vi "Get Graph.vi"(8 "error in (no error)":errorcluster, 11 "IV in":refnum<class "IV.lvclass">) -> (0 "error out":errorcluster, 1 "Y":dbl[](array[numeric]), 2 "X":dbl[](array[numeric]), 3 "IV out":refnum<class "IV.lvclass">, 4 "dY/dX":dbl[](array[numeric]))   [LabVIEW 2018, in "IV.lvclass"]
uses:
  IV.lvclass
  data/IV_data.lvclass
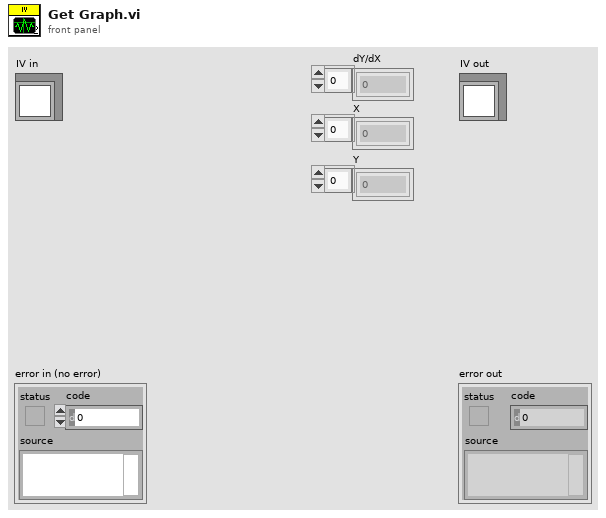
[diagram p1: front panel]
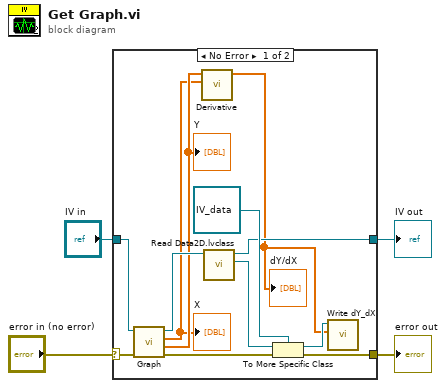
[diagram p0: block diagram]
diagram:
  n1 = case shown="No Error" "error in (no error)" {
    selector: "error in (no error)" -> [w14 w18]
    tunnel: [w6 w18] -> w3
    tunnel: [w10 w17] -> w1
    tunnel: "IV in" -> [w16 w17]
    frame No Error {
      n2 = call-dynamic "Graph.vi"("error in (no error)"=w14, "IV in"=w16) -> ("error out"=w15:errorcluster, "Y"=w9:dbl[], "X"=w8:dbl[], "IV out"=w13:refnum<class "IV.lvclass">)  [unwired: 6 in]
      "X" <- w8
      "Y" <- w9
      n3 = call "Derivative.vi"("X"=w8, "Y"=w9) -> ("dY/dX"=w5:dbl[])  [unwired: 9 in]
      "dY/dX" <- w5
      n4 = call-dynamic "Read Data2D.lvclass.vi"("Experiment2D in"=w13) -> ("Data2D.lvclass"=w12:refnum<class "Data2D.lvclass">, "Experiment2D out"=w10:refnum<class "IV.lvclass">)  [unwired: 8 in, 1 out]
      n5 = To More Specific Class(target class=refnum<class "IV_data.lvclass"> refnum ("IV_data.lvclass"), reference=w12, error in=w15) -> (specific class reference=w7:refnum<class "IV_data.lvclass">, error out=w6:errorcluster)
      n6 = call-dynamic "Write dY_dX.vi"("dY/dX"=w5, "IV_data in"=w7) -> ()  [unwired: 8 in, 2 out]
    }
    frame Error {
    }
  }
  "error out" <- w3
  "IV out" <- w1
